vi "Write Configuration File.vi"(8 "error in (no error)":errorcluster, 11 "Inst.TC in":refnum<class "Inst.TC.lvclass">) -> (0 "error out":errorcluster, 3 "Inst.TC out":refnum<class "Inst.TC.lvclass">)   [LabVIEW 2019, in "Inst.TC.lvclass"]
uses:
  Inst.TC.lvclass
  <userlib>/LevyLab/Configuration/Configuration.lvclass
  <userlib>/LevyLab/Instrument Framework/Instrument Types/VSource/Instrument.VSource.lvclass
  <userlib>/LevyLab/Instrument Framework/Instrument/Instrument.lvclass
  C:/Program Files (x86)/National Instruments/LabVIEW 2019/user.lib/LevyLab/Instrument Framework/Instrument Types/VSource/Instrument.VSource.lvclass
  C:/Program Files (x86)/National Instruments/LabVIEW 2019/user.lib/LevyLab/Instrument Framework/Instrument/Instrument.lvclass
  C:/Program Files (x86)/National Instruments/LabVIEW 2019/vi.lib/JKI/JKI SMO/SMO/SMO.lvclass
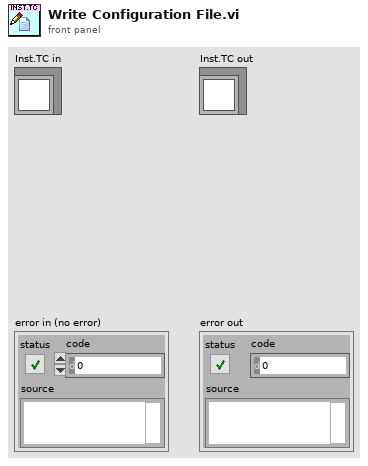
[diagram p1: front panel]
types:
  T1 = typedef "Inst.TC.lvclass/Inst.TC.Configuration--Cluster.ctl" = cluster{"LC Type":T2}
  T2 = typedef "Inst.TC.lvclass/Inst.TC.Type--Enum.ctl" = enum16{"CF.TC", "CF.TC.Z", "CF.FP", "MNK.TC", "MNK.TC.Z", "MNK.FP"}
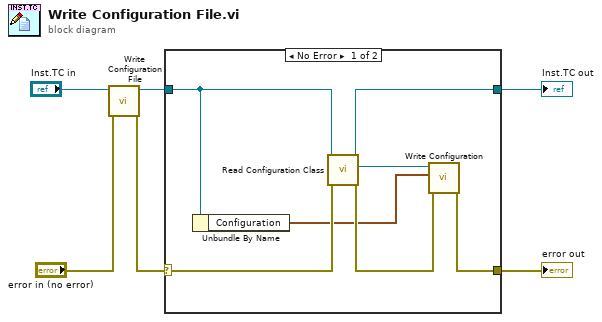
[diagram p0: block diagram]
diagram:
  n1 = call-parent "Write Configuration File.vi"("error in (no error)"="error in (no error)", "Instrument in"="Inst.TC in") -> ("error out"=w3:errorcluster, "Instrument out"=w1:refnum<class "Inst.TC.lvclass">)  [unwired: 8 in]
  n2 = case shown="No Error" w3 {
    selector: w3 -> [w9 w15]
    tunnel: w1 -> [w8 w14]
    tunnel: [w12 w14] -> w6
    tunnel: [w11 w15] -> w5
    frame No Error {
      n3 = Unbundle By Name(w8) -> ("Configuration"=w7:T1)
      n4 = call <userlib>:"Read Configuration Class.vi"("error in (no error)"=w9, "Instrument in"=w8) -> ("error out"=w13:errorcluster, "Configuration"=w10:refnum<class "Configuration.lvclass">, "Instrument out"=w12:refnum<class "Inst.TC.lvclass">)  [unwired: 7 in]
      n5 = call <userlib>:"Write Configuration.vi"("error in (no error)"=w13, "Variant"=w7, "Configuration in"=w10) -> ("error out"=w11:errorcluster)  [unwired: 7 in, 1 out]
    }
    frame Error {
    }
  }
  "Inst.TC out" <- w6
  "error out" <- w5
